vi "KeyDown Response.vi"(6 "PlatMods":T2, 8 "error in (no error)":errorcluster, 9 "VKey":T1, 10 "Char":i16, 11 "Editor Handler in":refnum<class "Listbox Handler.lvclass">) -> (0 "error out":errorcluster, 3 "Editor Handler out":refnum<class "Listbox Handler.lvclass">)   [LabVIEW 2017, in "Listbox Handler.lvclass"]
uses:
  Listbox Handler.lvclass
  C:/Program Files (x86)/National Instruments/LabVIEW 2017/vi.lib/LIEF/Image Editor Handler/Image Editor Handler.lvclass
  <vilib>/event_ctls.llb/eventvkey.ctl
  <vilib>/LIEF/Image Editor Handler/Image Editor Handler.lvclass/Image Editor Handler.ctl
  <vilib>/Utility/miscctls.llb/LVPoint32TypeDef.ctl
  Listbox Handler.lvclass/Listbox Handler.ctl
  <vilib>/LIEF/Image Editor Handler/Read Selected.vi
  <vilib>/LIEF/Image Editor Handler/Read Shapes.vi
  <vilib>/LIEF/Image Editor Handler/Read Renderer.vi
  <vilib>/LIEF/Image Editor Handler/Write Selected.vi
  <vilib>/LIEF/Image Editor Handler/Write Shapes.vi
  <vilib>/LIEF/Image Editor Handler/Write Renderer.vi
  <vilib>/LIEF/Forms/Shape/Shape.lvclass
  <vilib>/LIEF/Image/Image.lvclass
  <vilib>/LIEF/Image Editor Handler/Image Editor Handler.lvclass
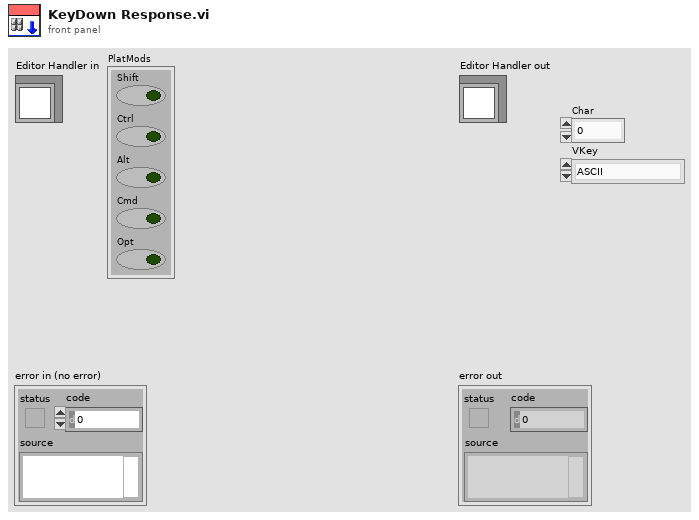
[diagram p1: front panel]
types:
  T1 = typedef "eventvkey.ctl" = enum16{"ASCII", "Enter", "Return", "Shift", "Ctrl", "Alt", "Cmd", "Opt", "Caps", "NumLock", "Clear", "Break", "Up", "Down", "Left", "Right", "Insert", "Delete", "Home", "End", "PageUp", "PageDown", "Escape", "Help", "Pause", "ScrollLock", "F1", "F2", "F3", "F4", "F5", "F6", "F7", "F8", "F9", "F10", "F11", "F12", "F13", "F14", "F15", "F16", "F17", "F18", "F19", "F20", "F21", "F22", "F23", "F24", "Play", "VolumeUp", "VolumeDown", "Mute", "Two Byte Char"}
  T2 = cluster{"Shift":bool, "Ctrl":bool, "Alt":bool, "Cmd":bool, "Opt":bool}
  T3 = typedef "LVPoint32TypeDef.ctl" = cluster{"Horizontal":i32, "Vertical":i32}
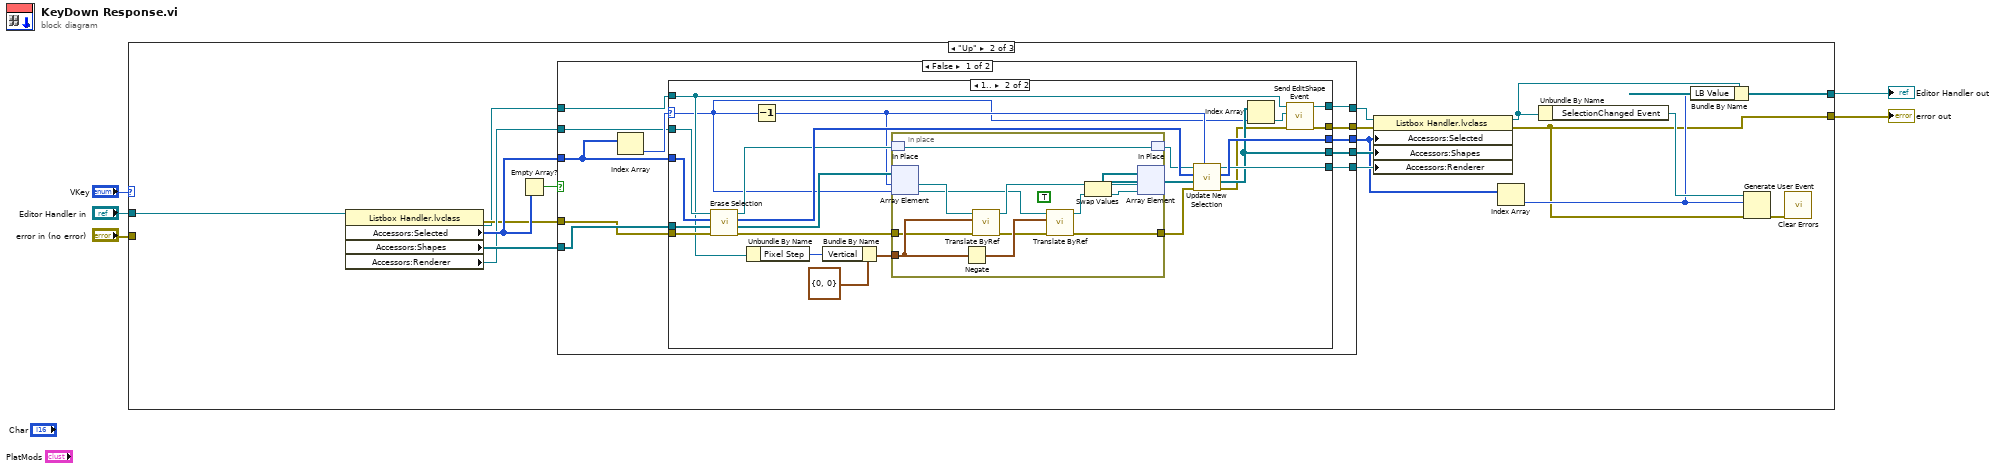
[diagram p0: block diagram]
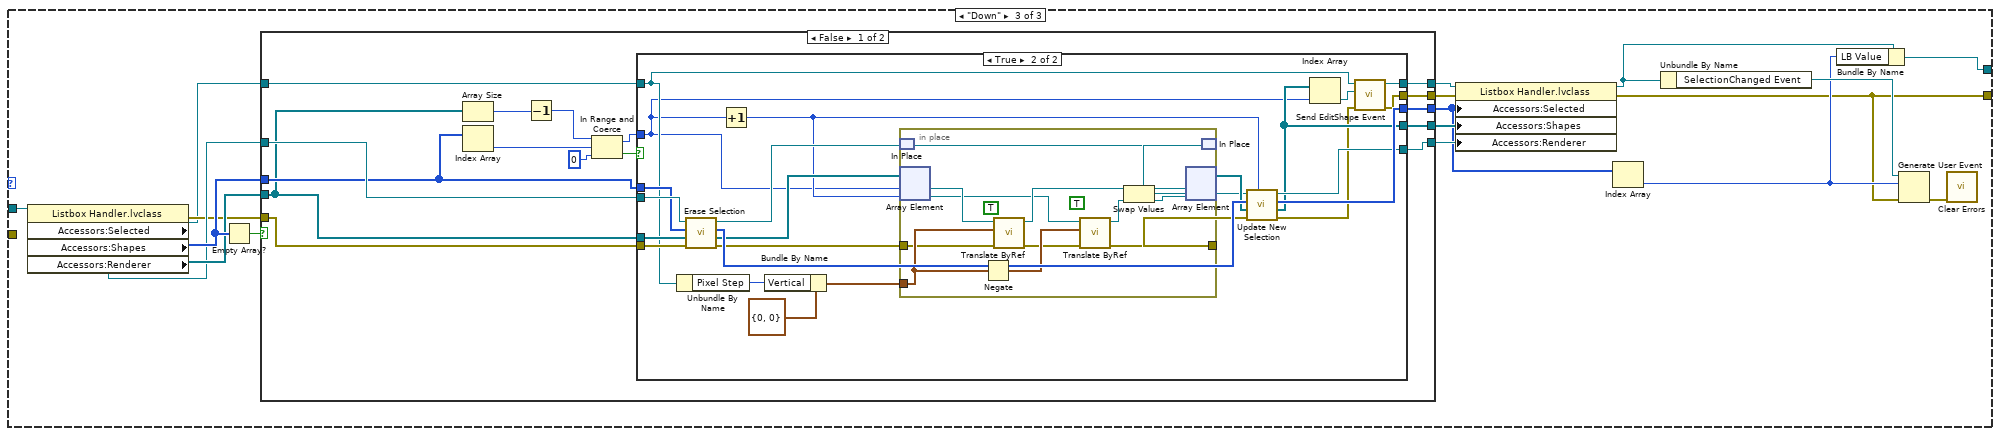
[diagram p5: hidden frame]
diagram:
  n1 = case shown="\"Up\"" "VKey" {
    tunnel: "Editor Handler in" -> [w7 w25 w100]
    tunnel: [w7 w12 w85] -> w2
    tunnel: [w6 w9 w83] -> w1
    tunnel: "error in (no error)" -> [w6 _ _]
    frame "ASCII", Default {
    }
    frame "Up" {
      n2 = property class="Listbox Handler.lvclass"(reference=w25) -> (reference out=w16:refnum<class "Listbox Handler.lvclass">, error out=w17:errorcluster, "Accessors:Selected"=w23:i16[], "Accessors:Shapes"=w22:refnum<data-value>[], "Accessors:Renderer"=w20:refnum<class "Image.lvclass">)  [unwired: 1 in]
      n3 = Empty Array?(array=w23) -> (empty?=w24:bool)
      n4 = case shown="False" w24 {
        tunnel: w23 -> [w33 w82]
        tunnel: [w36 w82] -> w14
        tunnel: w22 -> [w32 w81]
        tunnel: [w35 w81] -> w21
        tunnel: w20 -> [w31 w80]
        tunnel: [w30 w80] -> w19
        tunnel: [w29 w79] -> w18
        tunnel: w17 -> [w28 w79]
        tunnel: w16 -> [w27 w78]
        tunnel: [w26 w78] -> w15
        frame False {
          n5 = Index Array(array=w33) -> (element=w34:i16)  [unwired: 1 in]
          n6 = case shown="1.." w34 {
            selector: w34 -> [_ w42]
            tunnel: [w41 w61] -> w36
            tunnel: w32 -> [w40 w63]
            tunnel: [w40 w58] -> w35
            tunnel: w33 -> [w41 w64]
            tunnel: w31 -> [w39 w65]
            tunnel: [w39 w60] -> w30
            tunnel: [w38 w54] -> w29
            tunnel: w28 -> [w38 w59]
            tunnel: w27 -> [w37 w46]
            tunnel: [w37 w56] -> w26
            frame 0, Default {
            }
            frame 1.. {
              n7 = call <vilib>:"Erase Selection.vi"("error in (no error)"=w59, "Shape in"=w63, "Selected in"=w64, "Image in"=w65) -> ("error out"=w48:errorcluster, "Shape out"=w51:refnum<data-value>[], "Selected out"=w62:i16[], "Image out"=w53:refnum<class "Image.lvclass">)  [unwired: 4 in]
              n8 = Unbundle By Name(w46) -> ("Pixel Step"=w47:i32)
              n9 = Decrement(x=w42) -> (x-1=w43:i16)
              n10 = Bundle By Name(cluster=T3 {"Horizontal"=0, "Vertical"=0} ("Translation"), "Vertical"=w47) -> (w45:T3)
              n11 = in-place {
                in-place-border: w48 -> [w73]
                in-place-border: [w72] -> w49
                in-place-border: w45 -> [w76]
                (unwired) TRUE ("Force?")
                n12 = in-place-match #1(w53) -> (w77:refnum<class "Image.lvclass">)
                n13 = in-place-array #2(w51, w43, w42) -> (w69:refnum<data-value>, w67:refnum<data-value>)
                n14 = Negate(x=w76) -> (-x=w75:T3)
                n15 = call <vilib>:"Translate ByRef.vi"("error in (no error)"=w73, "Translation"=w76, "ShapeRef"=w69) -> ("error out"=w74:errorcluster, "ShapeRef Out"=w68:refnum<data-value>)  [unwired: 7 in]
                n16 = call <vilib>:"Translate ByRef.vi"("error in (no error)"=w74, "Translation"=w75, "ShapeRef"=w67) -> ("error out"=w72:errorcluster, "ShapeRef Out"=w66:refnum<data-value>)  [unwired: 7 in]
                n17 = Swap Values(12:w68, 14:w66) -> (1:w71:refnum<data-value>, 3:w70:refnum<data-value>)  [unwired: 1 in]
                n18 = in-place-array #2(w71, w70) -> (w50:refnum<data-value>[])  [unwired: 2 out]
                n19 = in-place-match #1(w77) -> (w52:refnum<class "Image.lvclass">)
              }
              n20 = call <vilib>:"Update New Selection.vi"("Node ID"=w43, "error in (no error)"=w49, "Shape in"=w50, "Selected in"=w62, "Image in"=w52) -> ("error out"=w55:errorcluster, "Shape out 2"=w58:refnum<data-value>[], "Selected out 2"=w61:i16[], "Image out"=w60:refnum<class "Image.lvclass">)  [unwired: 3 in]
              n21 = Index Array(array=w58, index=w42) -> (element=w57:refnum<data-value>)
              n22 = call <vilib>:"Send EditShape Event.vi"("error in (no error)"=w55, "Shape"=w57, "Editor Handler in"=w46) -> ("error out"=w54:errorcluster, "Editor Handler out"=w56:refnum<class "Listbox Handler.lvclass">)  [unwired: 7 in]
            }
          }
        }
        frame True {
        }
      }
      n23 = property class="Listbox Handler.lvclass"(reference=w15, error in=w18, "Accessors:Selected"=w14, "Accessors:Shapes"=w21, "Accessors:Renderer"=w19) -> (reference out=w8:refnum<class "Listbox Handler.lvclass">, error out=w9:errorcluster)
      n24 = Index Array(array=w14) -> (element=w10:i16)  [unwired: 1 in]
      n25 = Unbundle By Name(w8) -> ("SelectionChanged Event"=w13:refnum<user-event>)
      n26 = Bundle By Name(cluster=w8, "LB Value"=w10) -> (w12:refnum<class "Listbox Handler.lvclass">)
      n27 = Generate User Event(user event=w13, event data cluster=w10, error in=w9) -> (error out=w11:errorcluster)  [unwired: 1 in, 1 out]
      n28 = call <vilib>:"Clear Errors.vi"("error in (no error)"=w11) -> ()  [unwired: 5 in, 2 out]
    }
    frame "Down" {
      n29 = property class="Listbox Handler.lvclass"(reference=w100) -> (reference out=w91:refnum<class "Listbox Handler.lvclass">, error out=w92:errorcluster, "Accessors:Selected"=w98:i16[], "Accessors:Shapes"=w97:refnum<data-value>[], "Accessors:Renderer"=w95:refnum<class "Image.lvclass">)  [unwired: 1 in]
      n30 = Empty Array?(array=w98) -> (empty?=w99:bool)
      n31 = case shown="False" w99 {
        tunnel: w98 -> [w106 w162]
        tunnel: [w116 w162] -> w88
        tunnel: w97 -> [w101 w161]
        tunnel: [w115 w161] -> w96
        tunnel: w95 -> [w114 w160]
        tunnel: [w113 w160] -> w94
        tunnel: [w112 w159] -> w93
        tunnel: w92 -> [w111 w159]
        tunnel: w91 -> [w110 w158]
        tunnel: [w109 w158] -> w90
        frame False {
          n32 = Array Size(array=w101) -> (size(s)=w105:i32)
          n33 = Index Array(array=w106) -> (element=w108:i16)  [unwired: 1 in]
          n34 = Decrement(x=w105) -> (x-1=w104:i32)
          n35 = In Range and Coerce(upper limit=w104, x=w108, lower limit=0) -> (coerced(x)=w102:i32, In Range?=w103:bool)
          n36 = case shown="True" w103 {
            tunnel: [w121 w140] -> w116
            tunnel: w101 -> [w120 w143]
            tunnel: [w120 w132] -> w115
            tunnel: w106 -> [w121 w144]
            tunnel: w114 -> [w119 w145]
            tunnel: [w119 w138] -> w113
            tunnel: [w118 w127] -> w112
            tunnel: w111 -> [w118 w133]
            tunnel: w110 -> [w117 w126]
            tunnel: [w117 w129] -> w109
            tunnel: w102 -> [_ w123]
            frame False {
            }
            frame True {
              n37 = Unbundle By Name(w126) -> ("Pixel Step"=w122:i32)
              n38 = call <vilib>:"Erase Selection.vi"("error in (no error)"=w133, "Shape in"=w143, "Selected in"=w144, "Image in"=w145) -> ("error out"=w135:errorcluster, "Shape out"=w139:refnum<data-value>[], "Selected out"=w142:i16[], "Image out"=w137:refnum<class "Image.lvclass">)  [unwired: 4 in]
              n39 = Increment(x=w123) -> (x+1=w131:i32)
              n40 = Bundle By Name(cluster=T3 {"Horizontal"=0, "Vertical"=0} ("Translation"), "Vertical"=w122) -> (w124:T3)
              n41 = in-place {
                in-place-border: w135 -> [w153]
                in-place-border: [w152] -> w134
                in-place-border: w124 -> [w156]
                (unwired) TRUE ("Force?")
                (unwired) TRUE ("Force?")
                n42 = in-place-match #3(w137) -> (w157:refnum<class "Image.lvclass">)
                n43 = in-place-array #4(w139, w123, w131) -> (w149:refnum<data-value>, w147:refnum<data-value>)
                n44 = Negate(x=w156) -> (-x=w155:T3)
                n45 = call <vilib>:"Translate ByRef.vi"("error in (no error)"=w153, "Translation"=w156, "ShapeRef"=w149) -> ("error out"=w154:errorcluster, "ShapeRef Out"=w148:refnum<data-value>)  [unwired: 7 in]
                n46 = call <vilib>:"Translate ByRef.vi"("error in (no error)"=w154, "Translation"=w155, "ShapeRef"=w147) -> ("error out"=w152:errorcluster, "ShapeRef Out"=w146:refnum<data-value>)  [unwired: 7 in]
                n47 = Swap Values(12:w148, 14:w146) -> (1:w151:refnum<data-value>, 3:w150:refnum<data-value>)  [unwired: 1 in]
                n48 = in-place-array #4(w151, w150) -> (w141:refnum<data-value>[])  [unwired: 2 out]
                n49 = in-place-match #3(w157) -> (w136:refnum<class "Image.lvclass">)
              }
              n50 = call <vilib>:"Update New Selection.vi"("Node ID"=w131, "error in (no error)"=w134, "Shape in"=w141, "Selected in"=w142, "Image in"=w136) -> ("error out"=w128:errorcluster, "Shape out 2"=w132:refnum<data-value>[], "Selected out 2"=w140:i16[], "Image out"=w138:refnum<class "Image.lvclass">)  [unwired: 3 in]
              n51 = Index Array(array=w132, index=w123) -> (element=w130:refnum<data-value>)
              n52 = call <vilib>:"Send EditShape Event.vi"("error in (no error)"=w128, "Shape"=w130, "Editor Handler in"=w126) -> ("error out"=w127:errorcluster, "Editor Handler out"=w129:refnum<class "Listbox Handler.lvclass">)  [unwired: 7 in]
            }
          }
        }
        frame True {
        }
      }
      n53 = property class="Listbox Handler.lvclass"(reference=w90, error in=w93, "Accessors:Selected"=w88, "Accessors:Shapes"=w96, "Accessors:Renderer"=w94) -> (reference out=w86:refnum<class "Listbox Handler.lvclass">, error out=w83:errorcluster)
      n54 = Index Array(array=w88) -> (element=w84:i16)  [unwired: 1 in]
      n55 = Unbundle By Name(w86) -> ("SelectionChanged Event"=w87:refnum<user-event>)
      n56 = Bundle By Name(cluster=w86, "LB Value"=w84) -> (w85:refnum<class "Listbox Handler.lvclass">)
      n57 = Generate User Event(user event=w87, event data cluster=w84, error in=w83) -> (error out=w89:errorcluster)  [unwired: 1 in, 1 out]
      n58 = call <vilib>:"Clear Errors.vi"("error in (no error)"=w89) -> ()  [unwired: 5 in, 2 out]
    }
  }
  "error out" <- w1
  "Editor Handler out" <- w2
